vi "CowRow (SubVI).vi"(2 "OldVal":string[][](array[string]), 3 "NewVal in":string[][](array[string])) -> (0 "Col":i32, 1 "Row":i32)   [LabVIEW 2017]
panel:
  out "NewVal out":string[][](array[string])
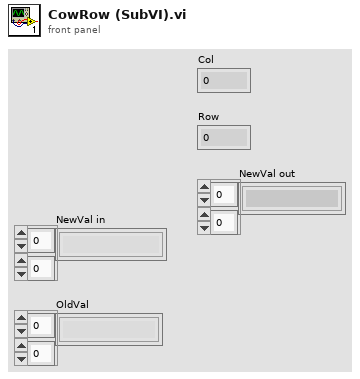
[diagram p1: front panel]
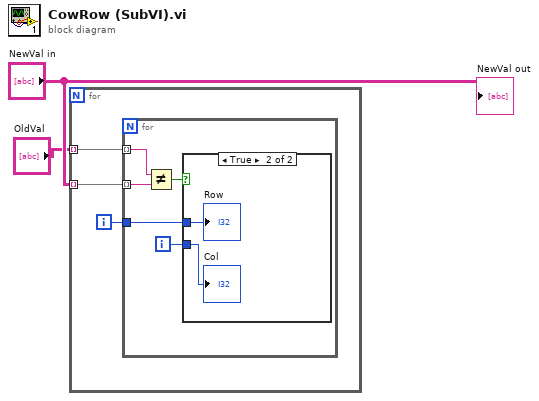
[diagram p0: block diagram]
diagram:
  n1 = for {
    tunnel: "OldVal" -> [w5] mode=indexing
    tunnel: "NewVal in" -> [w4] mode=indexing
    i -> [w3]
    n2 = for {
      tunnel: w5 -> [w10] mode=indexing
      tunnel: w4 -> [w9] mode=indexing
      tunnel: w3 -> [w6]
      i -> [w7]
      n3 = Not Equal?(x=w10, y=w9) -> (x != y?=w8:bool)
      n4 = case shown="True" w8 {
        tunnel: w7 -> [_ w11]
        tunnel: w6 -> [_ w12]
        frame False {
        }
        frame True {
          "Col" <- w11
          "Row" <- w12
        }
      }
    }
  }
  "NewVal out" <- "NewVal in"
